vi "Between 2 angles.vi"(8 "Test Angle":dbl, 10 "Angle 2":dbl, 11 "Angle 1":dbl) -> (3 "Is between Angle 1 and Angle 2":bool)   [LabVIEW 2011]
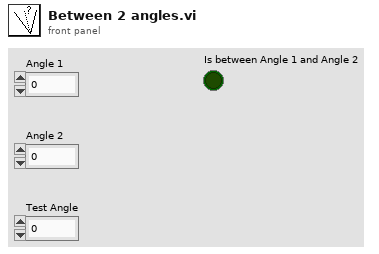
[diagram p1: front panel]
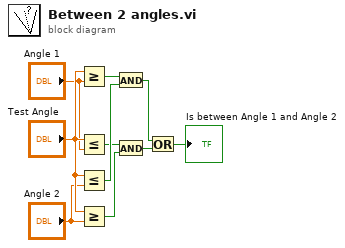
[diagram p0: block diagram]
diagram:
  n1 = Greater Or Equal?(x="Test Angle", y="Angle 1") -> (x >= y?=w10:bool)
  n2 = Less Or Equal?(x="Test Angle", y="Angle 1") -> (x <= y?=w8:bool)
  n3 = Less Or Equal?(x="Test Angle", y="Angle 2") -> (x <= y?=w9:bool)
  n4 = Greater Or Equal?(x="Test Angle", y="Angle 2") -> (x >= y?=w7:bool)
  n5 = And(x=w10, y=w9) -> (x .and. y?=w2:bool)
  n6 = And(x=w8, y=w7) -> (x .and. y?=w3:bool)
  n7 = Or(x=w2, y=w3) -> (x .or. y?=→"Is between Angle 1 and Angle 2":bool)
